vi "m10.wfg.04FM.vi"(1 "Param 0":dbl=1000.0, 2 "Param 1":dbl, 3 "Param 2":dbl, 4 "Param 3":dbl, 5 "error in (no error)":errorcluster, 8 "Waveform Properties":T1={"Fs (Hz)"=20000.0, "Amplitude (V)"=5.0, "Ramp (s)"=0.02} {"Ramp (s)" min=0.0; "Fs (Hz)" min=0.0}, 10 "Duration (s)":dbl=0.1) -> (14 "Waveform Out":waveform(dbl), 19 "error out":errorcluster)   [LabVIEW 2012]
panel:
  # "Start Frequency"
  # "End Frequency"
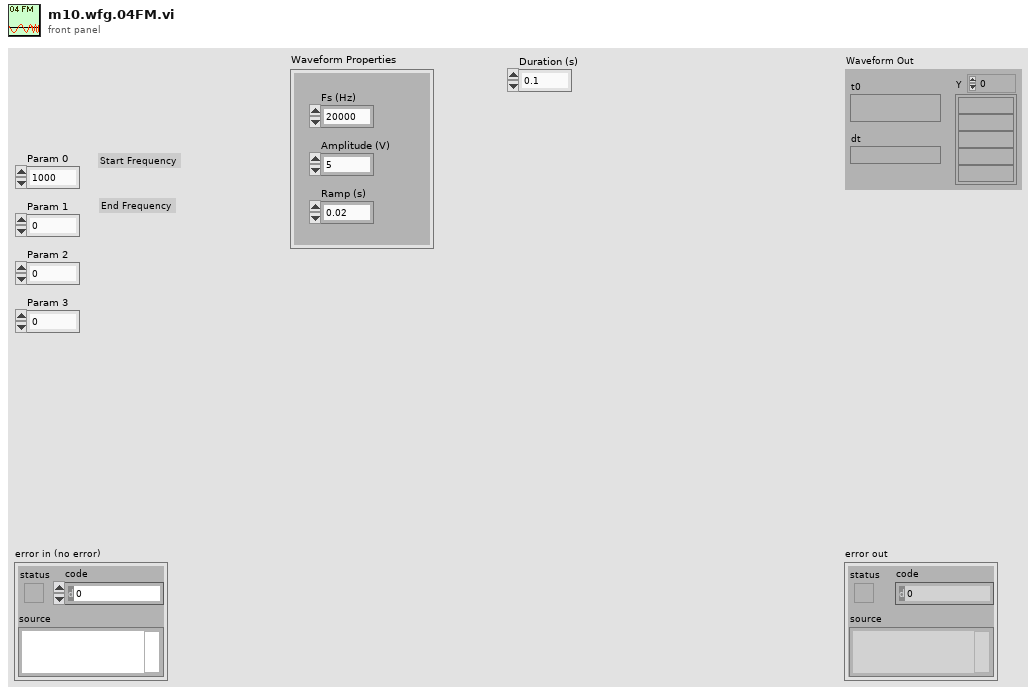
[diagram p1: front panel]
types:
  T1 = cluster{"Fs (Hz)":dbl, "Amplitude (V)":dbl, "Ramp (s)":dbl}
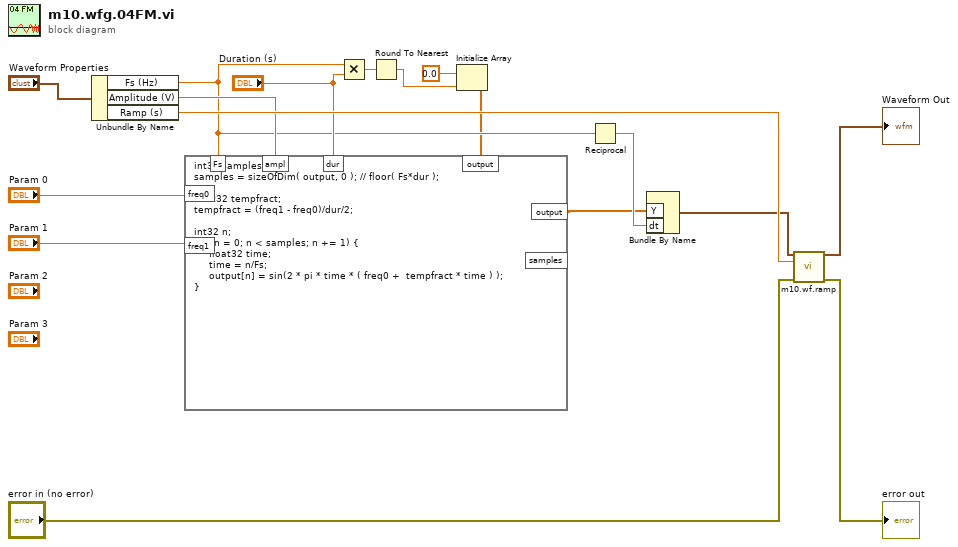
[diagram p0: block diagram]
diagram:
  n1 = Unbundle By Name("Waveform Properties") -> ("Fs (Hz)"=w5:dbl, "Amplitude (V)"=w11:dbl, "Ramp (s)"=w15:dbl)
  n2 = Multiply(x=w5, y="Duration (s)") -> (x*y=w4:dbl)
  n3 = Round To Nearest(number=w4) -> (nearest integer value=w3:dbl)
  n4 = Initialize Array(0.0 ("element"), w3) -> (w2:dbl[])
  n5 = formula code="int32 samples;\nsamples = sizeOfDim( output, 0 ); // floor( Fs*dur );\n\nfloat32 tempfract;\ntempfract = (freq1 - freq0)/dur/2;\n\nint32 n;\nfor( n = 0; n < samples; n += 1) {\n     float32 time;\n     time = n/Fs;\n     output[n] = sin(2 * pi * time * ( freq0 +  tempfract * time ) );\n}"("dur"="Duration (s)", "freq0"="Param 0", "freq1"="Param 1", "ampl"=w11, "Fs"=w5, "output"=w2) -> ("output"=w8:dbl[])  [unwired: 1 out]
  n6 = Reciprocal(x=w5) -> (1/x=w10:dbl)
  n7 = Bundle By Name("Y"=w8, "dt"=w10) -> (w9:waveform(dbl))  [unwired: 1 in]
  n8 = call "m10.wf.ramp.vi"("Waveform In"=w9, "Ramp Length (s)"=w15, "error in (no error)"="error in (no error)") -> ("Waveform Out"=→"Waveform Out":waveform(dbl), "error out"=→"error out":errorcluster)  [unwired: 11 in]
